vi "Read Error Count.vi"(11 "Test Case Result In":refnum<class "Test Case Result.lvclass">) -> (2 "Error count":i32, 3 "Test Case Result Out":refnum<class "Test Case Result.lvclass">)   [LabVIEW 2020, in "Test Case Result.lvclass"]
uses:
  Test Case Result.lvclass
  Assertion Result/Public/TypeDefs/Status.ctl
  Test Case Result.lvclass/Test Case Result.ctl
  Method Result/Method Result.lvclass/Method Result.ctl
  Method Result/Public/Read Status.vi
  Assertion Result/Assertion Result.lvclass
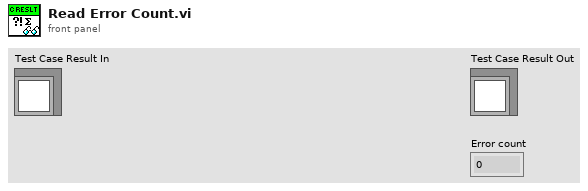
[diagram p1: front panel]
types:
  T1 = typedef "Assertion Result.lvclass/Status.ctl" = enum16{"Pass", "Fail", "Error", "Skipped", "Setup Error", "Broken", "Teardown Error"}
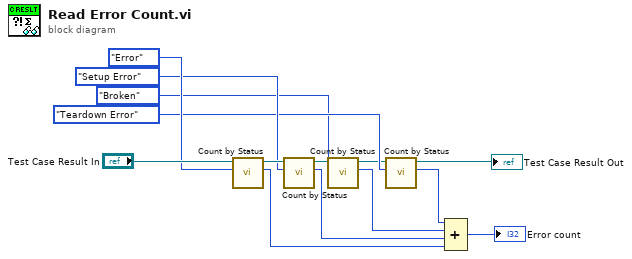
[diagram p0: block diagram]
diagram:
  n1 = call "Count by Status.vi"("Status"=Status."Error", "Test Case Result In"="Test Case Result In") -> ("Count"=w5:i32, "Test Case Result Out"=w13:refnum<class "Test Case Result.lvclass">)  [unwired: 8 in]
  n2 = call "Count by Status.vi"("Status"=Status."Setup Error", "Test Case Result In"=w13) -> ("Count"=w6:i32, "Test Case Result Out"=w4:refnum<class "Test Case Result.lvclass">)  [unwired: 8 in]
  n3 = call "Count by Status.vi"("Status"=Status."Broken", "Test Case Result In"=w4) -> ("Count"=w2:i32, "Test Case Result Out"=w3:refnum<class "Test Case Result.lvclass">)  [unwired: 8 in]
  n4 = call "Count by Status.vi"("Status"=Status."Teardown Error", "Test Case Result In"=w3) -> ("Count"=w7:i32, "Test Case Result Out"=→"Test Case Result Out":refnum<class "Test Case Result.lvclass">)  [unwired: 8 in]
  n5 = Compound Arithmetic op=ADD(w7, w2, w6, w5) -> (→"Error count":i32)
